vi "LOGGER Loop.vi"(8 "error in":errorcluster, 10 "Queues":T1, 11 "Notifiers":T2) -> (0 "error out":errorcluster)   [LabVIEW 2014, in "Logger.lvlib"]
uses:
  Logger.lvlib
  support/Message Queue/Message Queue.lvlib
  TypeDefs/Logger State.ctl
  TypeDefs/Logger Data.ctl
  Model/TypeDefs/Get Model Status Control.ctl
  Model/Model.lvlib
  <vilib>/ErrorRing/Error Ring.xnode
  support/Global names.vi
  <vilib>/Utility/error.llb/Error Cluster From Error Code.vi
  support/Message Queue/Message Cluster.ctl
  support/Notifiers/Notifiers.ctl
  Support/Notifiers/Notifiers.lvlib
  support/Message Queue/All Message Queues.ctl
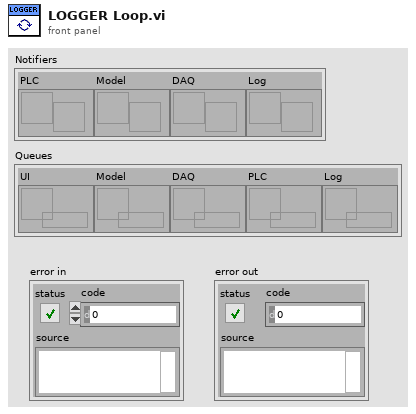
[diagram p1: front panel]
types:
  T1 = typedef "Message Queue.lvlib/All Message Queues.ctl" = cluster{"UI":refnum<queue>, "Model":refnum<queue>, "DAQ":refnum<queue>, "PLC":refnum<queue>, "Log":refnum<queue>}
  T2 = typedef "Notifiers.lvlib/Notifiers.ctl" = cluster{"PLC":refnum<notifier>, "Model":refnum<notifier>, "DAQ":refnum<notifier>, "Log":refnum<notifier>}
  T3 = typedef "Logger.lvlib/Logger Data.ctl" = cluster{"tdms file out":refnum<k34>, "State":T4, "Path":path}
  T4 = typedef "Logger.lvlib/Logger State.ctl" = enum16{"Idle", "Working"}
  T5 = typedef "Model.lvlib/Get Model Status Control.ctl" = cluster{"Position":dbl, "Pump State":bool, "Fluid Flow":dbl, "Fluid Level":dbl, "Barrel Number":i32, "Spill Alarm":bool, "Level Alarm":bool}
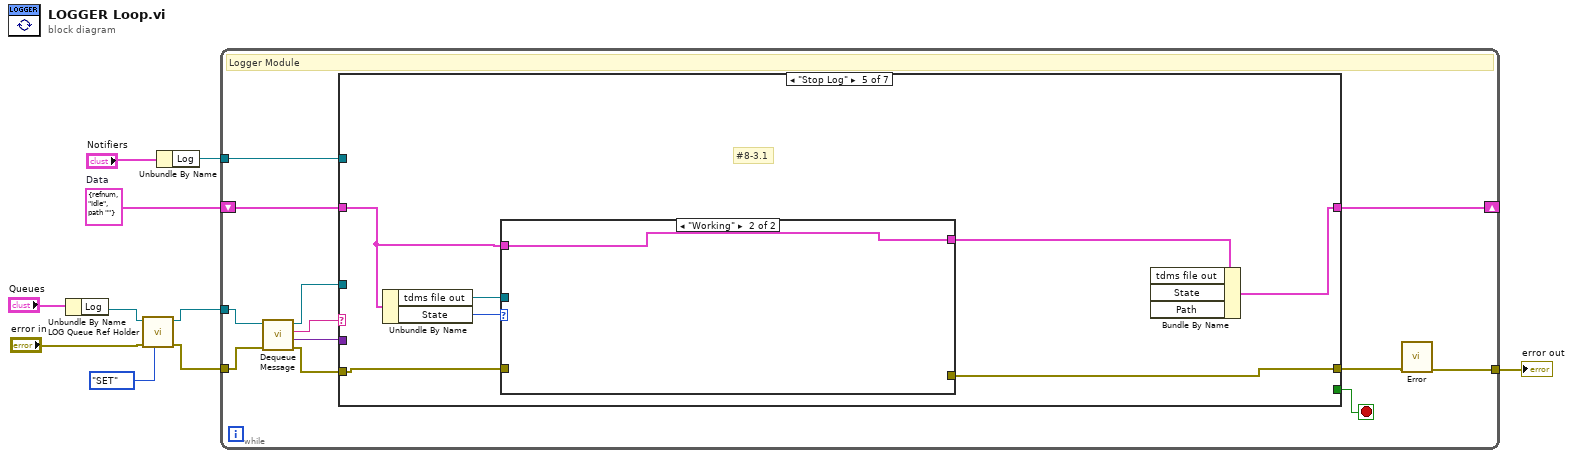
[diagram p0: block diagram]
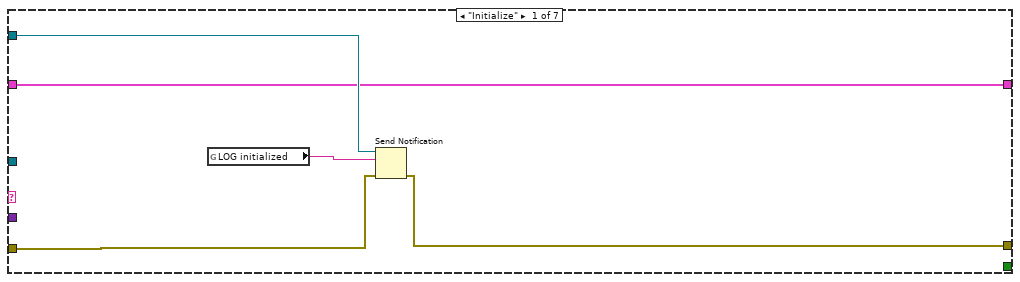
[diagram p2: hidden frame]
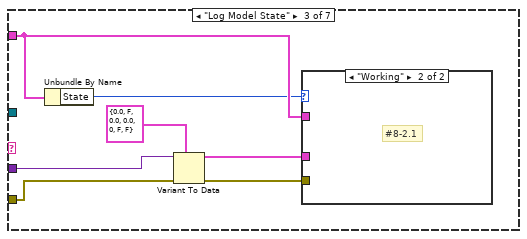
[diagram p4: hidden frame]
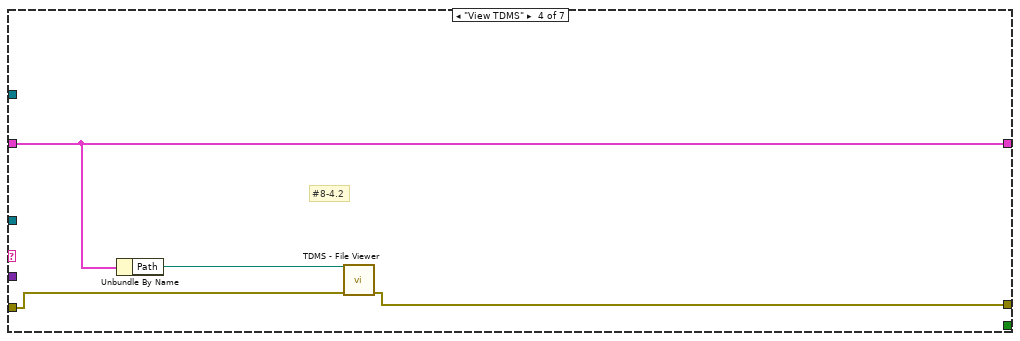
[diagram p6: hidden frame]
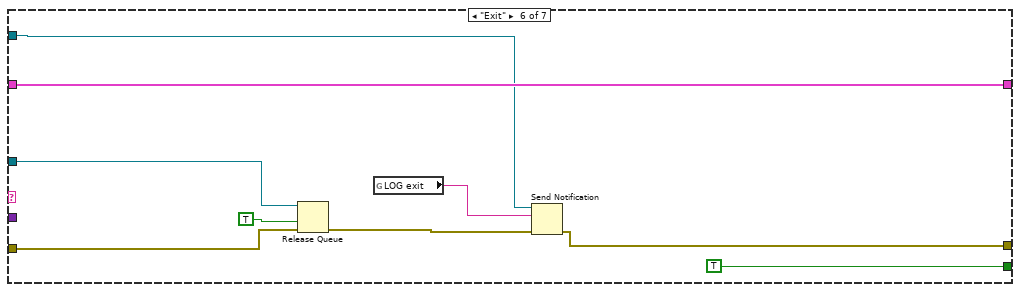
[diagram p8: hidden frame]
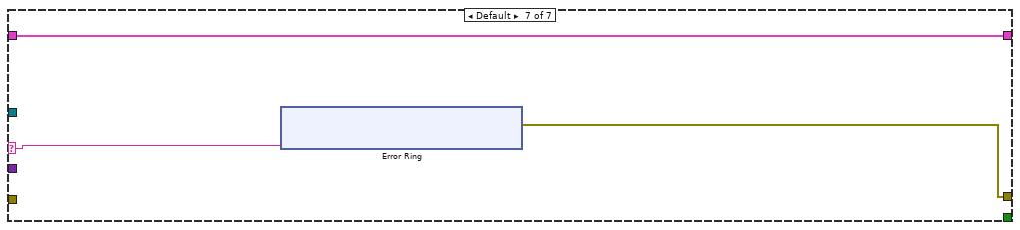
[diagram p9: hidden frame]
diagram:
  w10 = T3 {"tdms file out"=refnum, "State"=enum."Idle", "Path"=path ""}  # Data
  n1 = Unbundle By Name("Queues") -> ("Log"=w3:refnum<queue>)
  n2 = call "LOG Queue Ref Holder.vi"("Action"=enum16{"GET", "SET"}."SET", "error in"="error in", "Message Queue In"=w3) -> ("error out"=w4:errorcluster, "Input Message Queue"=w2:refnum<queue>)  [unwired: 7 in]
  n3 = Unbundle By Name("Notifiers") -> ("Log"=w6:refnum<notifier>)
  n4 = while {
    tunnel: w4 -> [w22]
    tunnel: w2 -> [w21]
    tunnel: [w11] -> w9
    shift-right: [w14] -> _
    shift-left: w10 -> [w15]
    tunnel: w6 -> [w13]
    stop <- w16 stop-if-true
    # "Logger Module"
    n5 = call "Dequeue Message.vi"("error in (no error)"=w22, "Message Queue"=w21) -> ("error out"=w20:errorcluster, "Message Data"=w17:variant, "Message"=w19:string, "dup Message Queue"=w18:refnum<queue>)  [unwired: 6 in]
    n6 = case shown="\"Stop Log\"" w19 {
      selector: w19 -> [_ _ _ _ _ _ w59]
      tunnel: w20 -> [w24 _ w34 w38 w43 w54 _]
      tunnel: w18 -> [_ _ _ _ _ w53 _]
      tunnel: w17 -> [_ _ w32 _ _ _ _]
      tunnel: [w25 _ _ w36 w39 w55 w58] -> w12
      tunnel: [_ _ _ _ _ TRUE _] -> w16
      tunnel: w15 -> [w26 _ w29 w37 w41 w57 w60]
      tunnel: [w26 _ _ w37 w45 w57 w60] -> w14
      tunnel: w13 -> [w27 _ _ _ _ w50 _]
      frame "Initialize" {
        n7 = global read "Global names.vi" "LOG initialized"() -> (w23:string)
        n8 = Send Notification(notification=w23, notifier=w27, error in (no error)=w24) -> (error out=w25:errorcluster)  [unwired: 1 out]
      }
      frame "Open Log" {
        # "#8-1.3"
      }
      frame "Log Model State" {
        n9 = Unbundle By Name(w29) -> ("State"=w28:T4)
        n10 = Variant To Data(error in=w34, type=T5 {"Position"=0.0, "Pump State"=FALSE, "Fluid Flow"=0.0, "Fluid Level"=0.0, "Barrel Number"=0, "Spill Alarm"=FALSE, "Level Alarm"=FALSE} ("Model Status"), Variant=w32) -> (data=w31:T5, error out=w30:errorcluster)
        n11 = case shown="\"Working\"" w28 {
          tunnel: w31 -> [_ _]
          tunnel: w30 -> [_ _]
          tunnel: w29 -> [_ _]
          frame Default {
          }
          frame "Working" {
            # "#8-2.1"
          }
        }
      }
      frame "View TDMS" {
        # "#8-4.2"
        n12 = Unbundle By Name(w37) -> ("Path"=w35:path)
        n13 = call <vilib>:"TDMS - File Viewer.vi"("error in (no error)"=w38, "file path"=w35) -> ("error out"=w36:errorcluster)  [unwired: 4 in, 1 out]
      }
      frame "Stop Log" {
        # "#8-3.1"
        n14 = Unbundle By Name(w41) -> ("tdms file out"=w44:refnum<k34>, "State"=w42:T4)
        n15 = case shown="\"Working\"" w42 {
          tunnel: w44 -> [_ _]
          tunnel: w43 -> [w47 _]
          tunnel: [w47 _] -> w39
          tunnel: w41 -> [w46 w48]
          tunnel: [w46 w48] -> w40
          frame "Idle", Default {
          }
          frame "Working" {
          }
        }
        n16 = Bundle By Name(cluster=w40) -> (w45:T3)  [unwired: 3 in]
      }
      frame "Exit" {
        n17 = Release Queue(queue=w53, force destroy? (F)=TRUE, error in (no error)=w54) -> (error out=w52:errorcluster)  [unwired: 2 out]
        n18 = global read "Global names.vi" "LOG exit"() -> (w49:string)
        n19 = Send Notification(notification=w49, notifier=w50, error in (no error)=w52) -> (error out=w55:errorcluster)  [unwired: 1 out]
      }
      frame Default {
        n20 = xnode "Error Ring"("parameter 0"=w59) -> ("error out"=w58:errorcluster)
      }
    }
    n21 = call "Error.vi"("error in"=w12) -> ("error out"=w11:errorcluster)  [unwired: 10 in]
  }
  "error out" <- w9
